vi "zad4.2_PH.vi"() -> ()   [LabVIEW 2023]
uses:
  <vilib>/Analysis/baseanly.llb/Mean (DBL).vi
  <vilib>/Analysis/NI_AALBase.lvlib
panel:
  out "Waveform Chart":dbl[](graph)=[0.9737991720980537, 0.3224651627768016, 0.43226203822087533, 0.27387365282913034, 0.3191576080947871]
  in  "Iloœæ iteracji":dbl=5.0
  out "œrednia":dbl=1.268760799781115
  out "minimum":dbl
  out "maksimum":dbl=0.7291667380409979
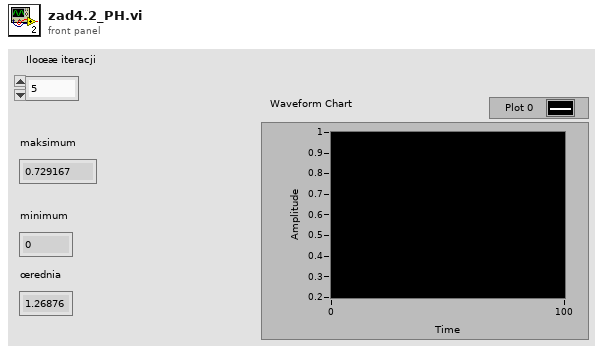
[diagram p1: front panel]
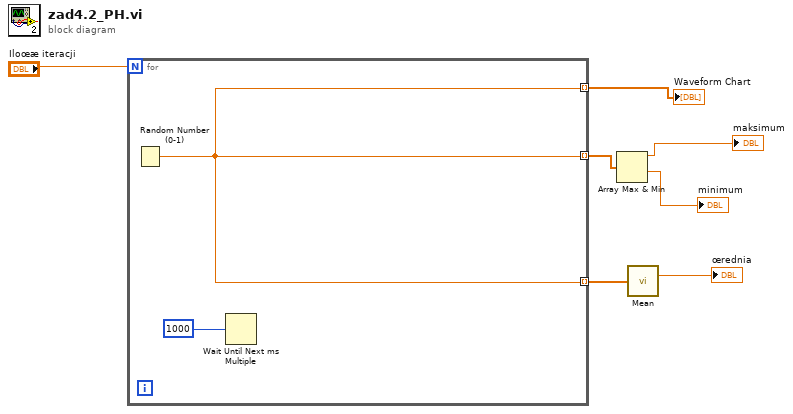
[diagram p0: block diagram]
diagram:
  n1 = for {
    N: "Iloœæ iteracji" -> [_]
    tunnel: [w8] -> w6 mode=indexing
    tunnel: [w8] -> w4 mode=indexing
    tunnel: [w8] -> w3 mode=indexing
    n2 = Random Number (0-1)() -> (number: 0 to 1=w8:dbl)
    n3 = Wait Until Next ms Multiple(millisecond multiple=1000) -> ()  [unwired: 1 out]
  }
  "Waveform Chart" <- w6
  n4 = Array Max & Min(array=w3) -> (max value=→"maksimum":dbl, min value=→"minimum":dbl)  [unwired: 2 out]
  n5 = call-poly <vilib>:"Mean.vi"("X"=w4) -> ("mean"=→"œrednia":dbl)  [unwired: 1 out]
